vi "Module - Alert Page.vi"() -> ()   [LabVIEW 2020]
uses:
  Control/State - eFGV.ctl
panel:
  out "Site Name":string="ALERT LIST"
  in  "Multicolumn Listbox":i32(listbox)
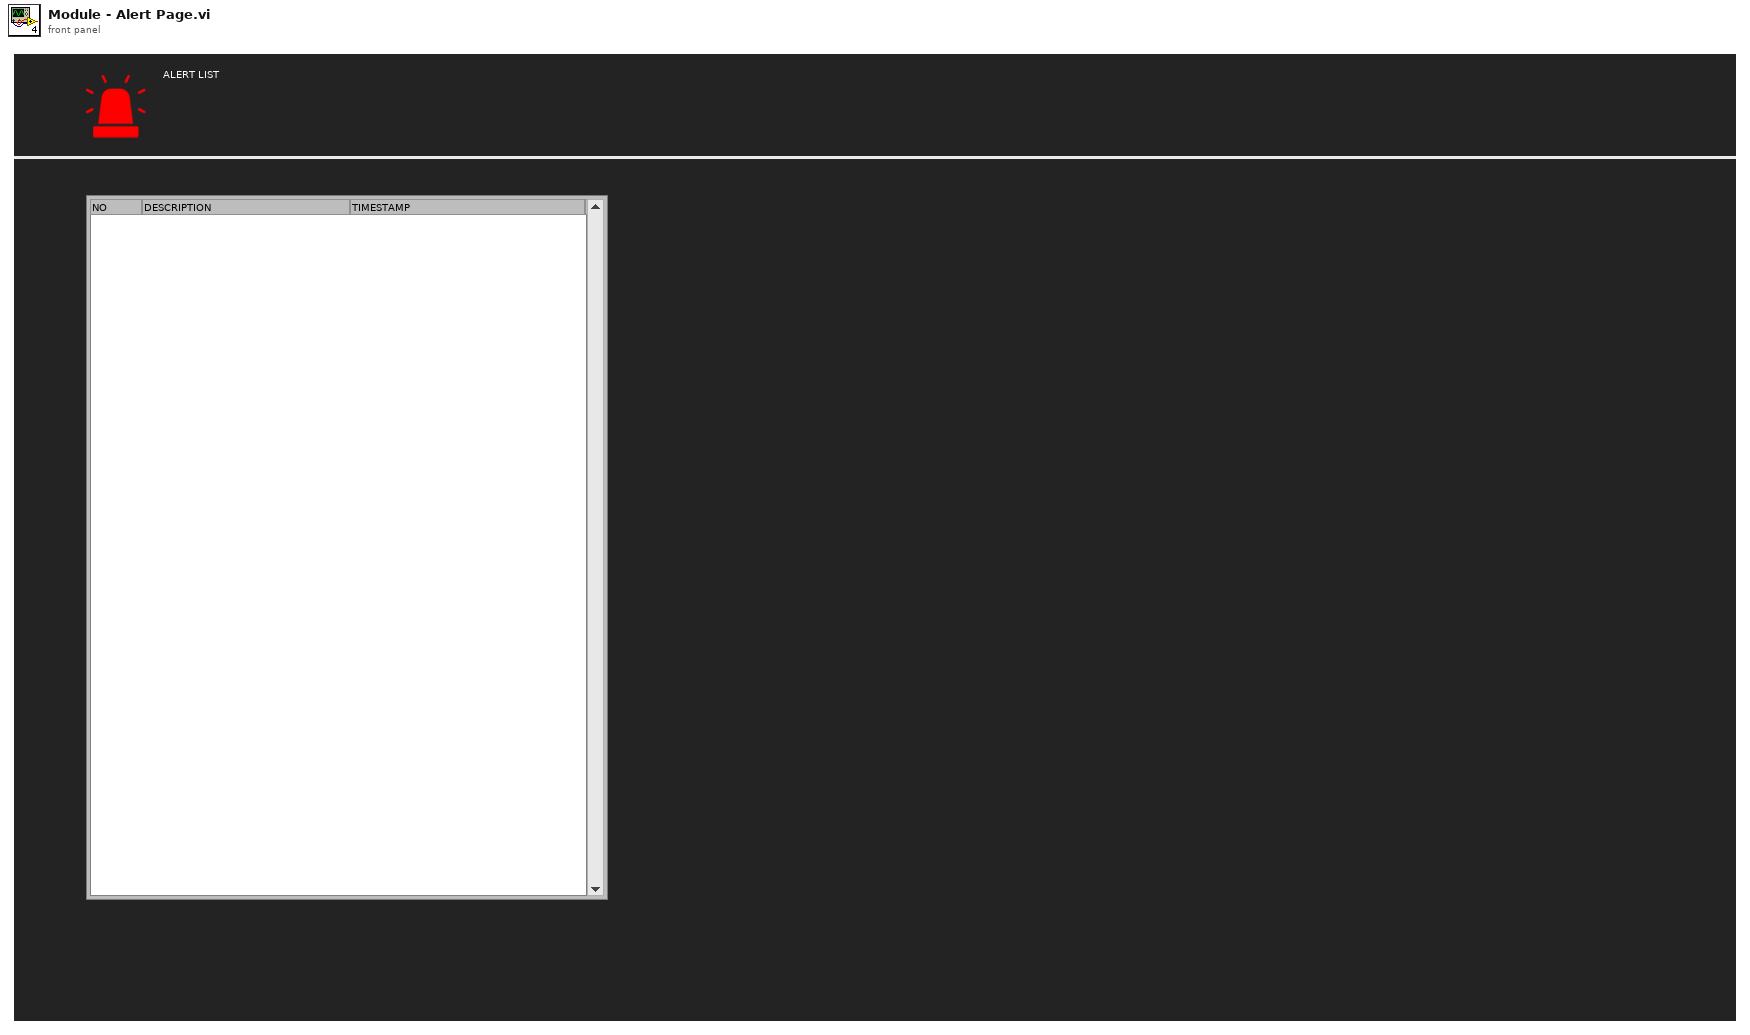
[diagram p1: front panel]
types:
  T1 = typedef "State - eFGV.ctl" = enum16{"Init", "Read", "Write", "Close"}
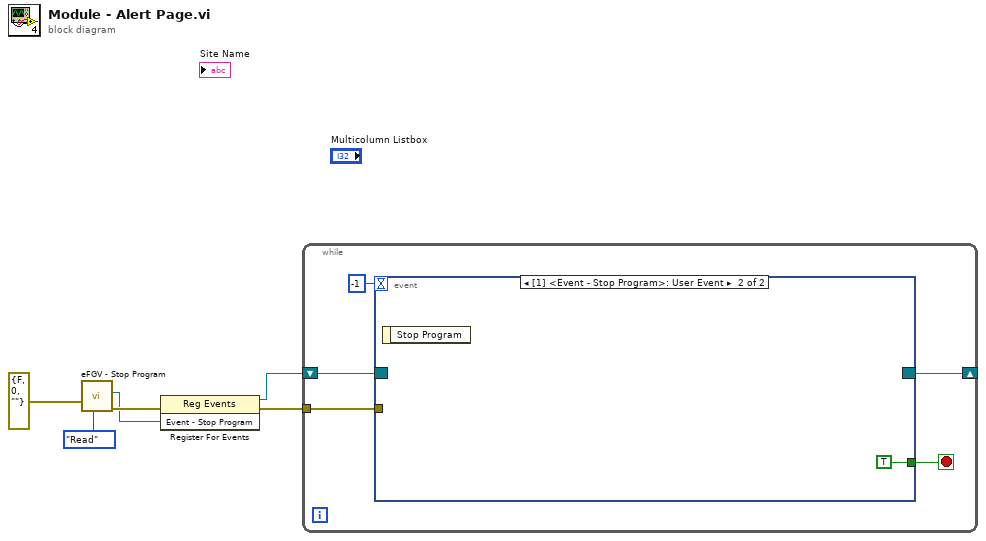
[diagram p0: block diagram]
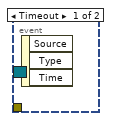
[diagram p2: hidden frame]
diagram:
  n1 = call "eFGV - Stop Program.vi"("State - eFGV"=State_-_eFGV."Read", "error in (no error)"=errorcluster {"status"=FALSE, "code"=0, "source"=""}) -> ("error out"=w5:errorcluster, "Event - Stop Program"=w4:refnum<user-event>)  [unwired: 8 in]
  n2 = register-events(error in=w5, w4) -> (reference out=w1:refnum<event-registration>, error out=w6:errorcluster)  [unwired: 1 in]
  n3 = while {
    tunnel: w6 -> [w10]
    shift-right: [w9] -> _
    shift-left: w1 -> [w11]
    stop <- w8 stop-if-true
    n4 = event shown="[1] <Event - Stop Program>: User Event" {
      selector: w11 -> [_ _]
      dyn-events: [_ _] -> w9
      timeout: -1 -> [_ _]
      tunnel: w10 -> [_ _]
      tunnel: [_ TRUE] -> w8
      event Timeout {
        n5 = event-data() -> ()  [unwired: 1 in, 3 out]
      }
      event User Event {
        n6 = event-data() -> ()  [unwired: 1 in, 1 out]
      }
    }
  }
